vi "property_contour_interval_read.vi"(4 "error in (no error)":errorcluster, 6 "Container State":T29, 7 "Display State In":T1={"Graph Properties"={"Projection Mode"=enum."Orthographic", "View Direction"=enum."Towards X-Y Plane", "Plot Area Color"=0, "Fast Draw"=FALSE, "X-Y"=FALSE, "Y-Z"=FALSE, "X-Z"=FALSE, "Lighting"=FALSE, "Refnum Queue"=refnum}, "Plot/Axes/Cursor Properties"={"Plot Properties Array"=[{"Projection Properties"={"Draw XY"=FALSE, "Draw YZ"=FALSE, "Draw XZ"=FALSE}, "Surface Properties"={"Draw surface"=TRUE, "Opacity"=1.0, "Shading"=TRUE, "Specular"=100, "Color Map"=[], "Interpolate Color"=TRUE, "Absolute Colormap"=TRUE}, "Contour Properties"={"Contour color"=0, "Axis"=enum."X", "Draw contour"=FALSE, "Antialias"=FALSE, "Line Width"=1.0, "Contour Line Style"=enum."Solid", "Mode"=enum."Levels", "Levels"=5.0, "Intervals"=1.0, "Anchored At"=0.0, "Anchored"=FALSE, "Level List"=[]}, "Normal Properties"={"Normal color"=0, "Normal Length"=0.0, "Normal Width"=0.0, "Draw Normal"=FALSE, "Antialiasing"=FALSE}, "Points/Lines Properties"={"Color"=0, "Antialiasing"=FALSE, "Point Size"=0.0, "Points / Lines"=enum."None", "Point Style"=enum."Point", "Line Style"=enum."Solid", "Line Width"=0.0}, "Plot ID"=0, "Coordinate System"=enum."Cartesian"}], "Value Pair Properties"={"X Value Pairs"={"Data Array"=[], "Show ticks"=FALSE, "Show grid lines"=FALSE, "Labels"=enum."Value"}, "Y Value Pairs"={"Data Array"=[], "Show ticks"=FALSE, "Show grid lines"=FALSE, "Labels"=enum."Value"}, "Z Value Pairs"={"Data Array"=[], "Show ticks"=FALSE, "Show grid lines"=FALSE, "Labels"=enum."Value"}}, "Axes Properties"={"Grid  Properties"={"Grid Visible"={"Draw X-grid"=FALSE, "Draw Y-grid"=FALSE, "Draw Z-grid"=FALSE}, "Grid Color"={"Color X"=0, "Color Y"=0, "Color Z"=0}}, "Ticks Properties"={"Minor Count"={"X"=0, "Y"=0, "Z"=0}, "Major Count"={"X"=0, "Y"=0, "Z"=0}, "Major Ticks Visible"={"X"=FALSE, "Y"=FALSE, "Z"=FALSE}, "Minor Ticks Visible"={"X"=FALSE, "Y"=FALSE, "Z"=FALSE}, "Tick Color"={"Color X"=0, "Color Y"=0, "Color Z"=0}}, "from/to cluster"={"X"={"Min"=0.0, "Max"=0.0}, "Y"={"Min"=0.0, "Max"=0.0}, "Z"={"Min"=0.0, "Max"=0.0}, "Amplitude"={"Min"=0.0, "Max"=0.0}}, "Caption Properties"={"Show Captions"={"Show X Caption"=FALSE, "Show Z Caption"=FALSE, "Show Y Caption"=FALSE, "Show Opposite X Caption"=FALSE, "Show Opposite Y Caption"=FALSE, "Show Opposite Z Caption"=FALSE}, "Captions"={"Caption X"="", "Caption Y"="", "Caption Z"=""}, "Caption Color"={"Color X"=0, "Color Y"=0, "Color Z"=0}, "Caption Font Size"={"Font Size X"=0, "Font Size Y"=0, "Font Size Z"=0}}, "Labels Properties"={"Label Visible"={"Show X Labels"=FALSE, "Show Y Labels"=FALSE, "Show Z Labels"=FALSE, "Show Opposite X Labels"=FALSE, "Show Opposite Y Labels"=FALSE, "Show Opposite Z Labels"=FALSE}, "Label Color"={"Color X"=0, "Color Y"=0, "Color Z"=0}, "Label Font Size"={"Font Size X"=0, "Font Size Y"=0, "Font Size Z"=0}}, "Auto Range On"={"X"=FALSE, "Y"=FALSE, "Z"=FALSE}}, "Cursor Properties Array"=[], "Format strings"={"XAxis"="", "YAxis"="", "ZAxis"=""}, "Lighting Properties"={"Brightness"=0, "Focus"=0.0, "Linear Attenuation"=0.0, "Quadratic Attenuation"=0.0}, "Lights"=[]}, "Active Plot"=0, "Active Axis"=0, "Active Cursor"=0, "Disable Updates"=FALSE}) -> (0 "error out":errorcluster, 2 "Value":sgl, 3 "Display State Out":T1={"Graph Properties"={"Projection Mode"=enum."Orthographic", "View Direction"=enum."Towards X-Y Plane", "Plot Area Color"=0, "Fast Draw"=FALSE, "X-Y"=FALSE, "Y-Z"=FALSE, "X-Z"=FALSE, "Lighting"=FALSE, "Refnum Queue"=refnum}, "Plot/Axes/Cursor Properties"={"Plot Properties Array"=[{"Projection Properties"={"Draw XY"=FALSE, "Draw YZ"=FALSE, "Draw XZ"=FALSE}, "Surface Properties"={"Draw surface"=TRUE, "Opacity"=1.0, "Shading"=TRUE, "Specular"=100, "Color Map"=[], "Interpolate Color"=TRUE, "Absolute Colormap"=TRUE}, "Contour Properties"={"Contour color"=0, "Axis"=enum."X", "Draw contour"=FALSE, "Antialias"=FALSE, "Line Width"=1.0, "Contour Line Style"=enum."Solid", "Mode"=enum."Levels", "Levels"=5.0, "Intervals"=1.0, "Anchored At"=0.0, "Anchored"=FALSE, "Level List"=[]}, "Normal Properties"={"Normal color"=0, "Normal Length"=0.0, "Normal Width"=0.0, "Draw Normal"=FALSE, "Antialiasing"=FALSE}, "Points/Lines Properties"={"Color"=0, "Antialiasing"=FALSE, "Point Size"=0.0, "Points / Lines"=enum."None", "Point Style"=enum."Point", "Line Style"=enum."Solid", "Line Width"=0.0}, "Plot ID"=0, "Coordinate System"=enum."Cartesian"}], "Value Pair Properties"={"X Value Pairs"={"Data Array"=[], "Show ticks"=FALSE, "Show grid lines"=FALSE, "Labels"=enum."Value"}, "Y Value Pairs"={"Data Array"=[], "Show ticks"=FALSE, "Show grid lines"=FALSE, "Labels"=enum."Value"}, "Z Value Pairs"={"Data Array"=[], "Show ticks"=FALSE, "Show grid lines"=FALSE, "Labels"=enum."Value"}}, "Axes Properties"={"Grid  Properties"={"Grid Visible"={"Draw X-grid"=FALSE, "Draw Y-grid"=FALSE, "Draw Z-grid"=FALSE}, "Grid Color"={"Color X"=0, "Color Y"=0, "Color Z"=0}}, "Ticks Properties"={"Minor Count"={"X"=0, "Y"=0, "Z"=0}, "Major Count"={"X"=0, "Y"=0, "Z"=0}, "Major Ticks Visible"={"X"=FALSE, "Y"=FALSE, "Z"=FALSE}, "Minor Ticks Visible"={"X"=FALSE, "Y"=FALSE, "Z"=FALSE}, "Tick Color"={"Color X"=0, "Color Y"=0, "Color Z"=0}}, "from/to cluster"={"X"={"Min"=0.0, "Max"=0.0}, "Y"={"Min"=0.0, "Max"=0.0}, "Z"={"Min"=0.0, "Max"=0.0}, "Amplitude"={"Min"=0.0, "Max"=0.0}}, "Caption Properties"={"Show Captions"={"Show X Caption"=FALSE, "Show Z Caption"=FALSE, "Show Y Caption"=FALSE, "Show Opposite X Caption"=FALSE, "Show Opposite Y Caption"=FALSE, "Show Opposite Z Caption"=FALSE}, "Captions"={"Caption X"="", "Caption Y"="", "Caption Z"=""}, "Caption Color"={"Color X"=0, "Color Y"=0, "Color Z"=0}, "Caption Font Size"={"Font Size X"=0, "Font Size Y"=0, "Font Size Z"=0}}, "Labels Properties"={"Label Visible"={"Show X Labels"=FALSE, "Show Y Labels"=FALSE, "Show Z Labels"=FALSE, "Show Opposite X Labels"=FALSE, "Show Opposite Y Labels"=FALSE, "Show Opposite Z Labels"=FALSE}, "Label Color"={"Color X"=0, "Color Y"=0, "Color Z"=0}, "Label Font Size"={"Font Size X"=0, "Font Size Y"=0, "Font Size Z"=0}}, "Auto Range On"={"X"=FALSE, "Y"=FALSE, "Z"=FALSE}}, "Cursor Properties Array"=[], "Format strings"={"XAxis"="", "YAxis"="", "ZAxis"=""}, "Lighting Properties"={"Brightness"=0, "Focus"=0.0, "Linear Attenuation"=0.0, "Quadratic Attenuation"=0.0}, "Lights"=[]}, "Active Plot"=0, "Active Axis"=0, "Active Cursor"=0, "Disable Updates"=FALSE})   [LabVIEW 2020, in "3DPC_SurfacePlot.xctl"]
uses:
  <vilib>/Native 3D Graph/xcontrol/3DPC_SurfacePlot.xctl
  <vilib>/_xctls/Container State.ctl
  <vilib>/Native 3D Graph/xcontrol/State.ctl
  <vilib>/Native 3D Graph/typedefs/prop_graph.ctl
  <vilib>/Native 3D Graph/typedefs/all_non_graph_prop.ctl
  <vilib>/Native 3D Graph/typedefs/prop_plot_all_array.ctl
  <vilib>/Native 3D Graph/typedefs/prop_plot_all.ctl
  <vilib>/Native 3D Graph/typedefs/prop_plot_projection.ctl
  <vilib>/Native 3D Graph/typedefs/prop_plot_surface.ctl
  <vilib>/Native 3D Graph/typedefs/prop_plot_contour.ctl
  <vilib>/Native 3D Graph/typedefs/prop_plot_normal.ctl
  <vilib>/Native 3D Graph/typedefs/prop_plot_point_line.ctl
  <vilib>/Native 3D Graph/typedefs/prop_value_pair_all.ctl
  <vilib>/Native 3D Graph/typedefs/prop_value_pair_1d.ctl
  <vilib>/Native 3D Graph/typedefs/prop_axes_all.ctl
  <vilib>/Native 3D Graph/typedefs/prop_axes_grid.ctl
  <vilib>/Native 3D Graph/typedefs/prop_axes_ticks.ctl
  <vilib>/Native 3D Graph/typedefs/range_cluster.ctl
  <vilib>/Native 3D Graph/typedefs/min_max.ctl
  <vilib>/Native 3D Graph/typedefs/prop_axes_captions.ctl
  <vilib>/Native 3D Graph/typedefs/prop_axes_labels.ctl
  <vilib>/Native 3D Graph/typedefs/prop_axes_autorange.ctl
  <vilib>/Native 3D Graph/typedefs/prop_cursor_all_array.ctl
  <vilib>/Native 3D Graph/typedefs/prop_cursor_point.ctl
  <vilib>/Native 3D Graph/typedefs/prop_cursor_position.ctl
  <vilib>/Native 3D Graph/typedefs/prop_cursor_line.ctl
  <vilib>/Native 3D Graph/typedefs/prop_cursor_plane.ctl
  <vilib>/Native 3D Graph/typedefs/prop_cursor_text.ctl
  <vilib>/Native 3D Graph/typedefs/prop_format.ctl
  <vilib>/Native 3D Graph/typedefs/prop_lighting.ctl
  <vilib>/_xctls/XControlSupport.lvlib
panel:
  # "Replace the Value Indicator below with an Indicator of desired type.\nDo not remove this Indicator or the others from the connector pane. \nDo not change the connector pane pattern.\nThe Value Indicator should always be the second terminal from top on the output side in the connector pane."
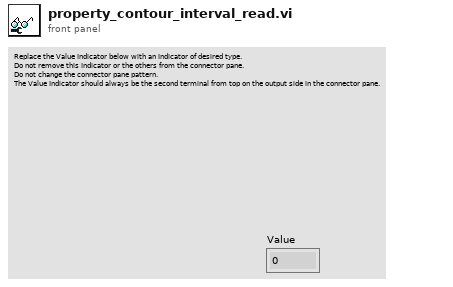
[diagram p1: front panel]
types:
  T1 = typedef "3DPC_SurfacePlot.xctl/State.ctl" = cluster{"Graph Properties":T2, "Plot/Axes/Cursor Properties":T3, "Active Plot":i32, "Active Axis":i32, "Active Cursor":i32, "Disable Updates":bool}
  T2 = typedef "3DPC_SurfacePlot.xctl/prop_graph.ctl" = cluster{"Projection Mode":enum16{"Orthographic", "Perspective"}, "View Direction":enum32{"Towards X-Y Plane", "Towards Y-Z Plane", "Towards X-Z Plane", "User Define"}, "Plot Area Color":u32, "Fast Draw":bool, "X-Y":bool, "Y-Z":bool, "X-Z":bool, "Lighting":bool, "Refnum Queue":refnum<queue>}
  T3 = typedef "3DPC_SurfacePlot.xctl/all_non_graph_prop.ctl" = cluster{"Plot Properties Array":T4, "Value Pair Properties":T11, "Axes Properties":T13, "Cursor Properties Array":T21, "Format strings":T27, "Lighting Properties":T28, "Lights":cluster{"Position":cluster{"X":sgl, "Y":sgl, "Z":sgl}, "Direction":cluster{"X":sgl, "Y":sgl, "Z":sgl}}[]}
  T4 = typedef "3DPC_SurfacePlot.xctl/prop_plot_all_array.ctl" = T5[]
  T5 = typedef "3DPC_SurfacePlot.xctl/prop_plot_all.ctl" = cluster{"Projection Properties":T6, "Surface Properties":T7, "Contour Properties":T8, "Normal Properties":T9, "Points/Lines Properties":T10, "Plot ID":i32, "Coordinate System":enum16{"Cartesian", "Cylindrical", "Spherical"}}
  T6 = typedef "3DPC_SurfacePlot.xctl/prop_plot_projection.ctl" = cluster{"Draw XY":bool, "Draw YZ":bool, "Draw XZ":bool}
  T7 = typedef "3DPC_SurfacePlot.xctl/prop_plot_surface.ctl" = cluster{"Draw surface":bool, "Opacity":dbl, "Shading":bool, "Specular":i32, "Color Map":cluster{dbl, u32}[], "Interpolate Color":bool, "Absolute Colormap":bool}
  T8 = typedef "3DPC_SurfacePlot.xctl/prop_plot_contour.ctl" = cluster{"Contour color":u32, "Axis":enum16{"X", "Y", "Z"}, "Draw contour":bool, "Antialias":bool, "Line Width":sgl, "Contour Line Style":enum16{"Solid", "Dash", "Dot", "Dash Dot"}, "Mode":enum16{"Levels", "Intervals", "Level List"}, "Levels":sgl, "Intervals":sgl, "Anchored At":sgl, "Anchored":bool, "Level List":dbl[]}
  T9 = typedef "3DPC_SurfacePlot.xctl/prop_plot_normal.ctl" = cluster{"Normal color":u32, "Normal Length":sgl, "Normal Width":sgl, "Draw Normal":bool, "Antialiasing":bool}
  T10 = typedef "3DPC_SurfacePlot.xctl/prop_plot_point_line.ctl" = cluster{"Color":u32, "Antialiasing":bool, "Point Size":sgl, "Points / Lines":enum16{"None", "Points", "Lines", "Both"}, "Point Style":enum16{"Point", "EmptySquare", "Asterisk", "Diamond", "EmptyCircle", "Circle", "X"}, "Line Style":enum16{"Solid", "Dash", "Dot", "Dash Dot"}, "Line Width":sgl}
  T11 = typedef "3DPC_SurfacePlot.xctl/prop_value_pair_all.ctl" = cluster{"X Value Pairs":cluster{"Data Array":cluster{"Value":sgl, "Index":i32, "Name":string}[], "Show ticks":bool, "Show grid lines":bool, "Labels":enum16{"Value", "None", "Name"}}, "Y Value Pairs":T12, "Z Value Pairs":T12}
  T12 = typedef "3DPC_SurfacePlot.xctl/prop_value_pair_1d.ctl" = cluster{"Data Array":cluster{"Value":sgl, "Index":i32, "Name":string}[], "Show ticks":bool, "Show grid lines":bool, "Labels":enum16{"Value", "None", "Name"}}
  T13 = typedef "3DPC_SurfacePlot.xctl/prop_axes_all.ctl" = cluster{"Grid  Properties":T14, "Ticks Properties":T15, "from/to cluster":T16, "Caption Properties":T18, "Labels Properties":T19, "Auto Range On":T20}
  T14 = typedef "3DPC_SurfacePlot.xctl/prop_axes_grid.ctl" = cluster{"Grid Visible":cluster{"Draw X-grid":bool, "Draw Y-grid":bool, "Draw Z-grid":bool}, "Grid Color":cluster{"Color X":u32, "Color Y":u32, "Color Z":u32}}
  T15 = typedef "3DPC_SurfacePlot.xctl/prop_axes_ticks.ctl" = cluster{"Minor Count":cluster{"X":i32, "Y":i32, "Z":i32}, "Major Count":cluster{"X":i32, "Y":i32, "Z":i32}, "Major Ticks Visible":cluster{"X":bool, "Y":bool, "Z":bool}, "Minor Ticks Visible":cluster{"X":bool, "Y":bool, "Z":bool}, "Tick Color":cluster{"Color X":u32, "Color Y":u32, "Color Z":u32}}
  T16 = typedef "3DPC_SurfacePlot.xctl/range_cluster.ctl" = cluster{"X":T17, "Y":T17, "Z":T17, "Amplitude":T17}
  T17 = typedef "3DPC_SurfacePlot.xctl/min_max.ctl" = cluster{"Min":sgl, "Max":sgl}
  T18 = typedef "3DPC_SurfacePlot.xctl/prop_axes_captions.ctl" = cluster{"Show Captions":cluster{"Show X Caption":bool, "Show Z Caption":bool, "Show Y Caption":bool, "Show Opposite X Caption":bool, "Show Opposite Y Caption":bool, "Show Opposite Z Caption":bool}, "Captions":cluster{"Caption X":string, "Caption Y":string, "Caption Z":string}, "Caption Color":cluster{"Color X":u32, "Color Y":u32, "Color Z":u32}, "Caption Font Size":cluster{"Font Size X":i16, "Font Size Y":i16, "Font Size Z":i16}}
  T19 = typedef "3DPC_SurfacePlot.xctl/prop_axes_labels.ctl" = cluster{"Label Visible":cluster{"Show X Labels":bool, "Show Y Labels":bool, "Show Z Labels":bool, "Show Opposite X Labels":bool, "Show Opposite Y Labels":bool, "Show Opposite Z Labels":bool}, "Label Color":cluster{"Color X":u32, "Color Y":u32, "Color Z":u32}, "Label Font Size":cluster{"Font Size X":i16, "Font Size Y":i16, "Font Size Z":i16}}
  T20 = typedef "3DPC_SurfacePlot.xctl/prop_axes_autorange.ctl" = cluster{"X":bool, "Y":bool, "Z":bool}
  T21 = typedef "3DPC_SurfacePlot.xctl/prop_cursor_all_array.ctl" = cluster{"Cursor Visible":bool, "Cursor Enable":bool, "Cursor Point":T22, "Cursor Position":T23, "Cursor Line":T24, "Cursor Plane":T25, "Cursor Name":string, "Cursor Text":T26}[]
  T22 = typedef "3DPC_SurfacePlot.xctl/prop_cursor_point.ctl" = cluster{"Point Color":u32, "Point Size":dbl, "Point Visible":bool}
  T23 = typedef "3DPC_SurfacePlot.xctl/prop_cursor_position.ctl" = cluster{"Position X":dbl, "Position Y":dbl, "Position Z":dbl, "Position Snap To":enum16{"Fixed", "Nearest Plot", "Snap to Plot"}, "Polsition Pick Plot":u16, "Position Column":i32, "Position Row":i32}
  T24 = typedef "3DPC_SurfacePlot.xctl/prop_cursor_line.ctl" = cluster{"Line Color":u32, "Line Width":dbl, "Line Visible":bool}
  T25 = typedef "3DPC_SurfacePlot.xctl/prop_cursor_plane.ctl" = cluster{"Plane Opacity":dbl, "Plane Color":u32, "Plane YZ":bool, "Plane XZ":bool, "Plane XY":bool}
  T26 = typedef "3DPC_SurfacePlot.xctl/prop_cursor_text.ctl" = cluster{"Cursor Name":string, "Font Size":i32, "Show Position":bool, "Show Name":bool, "Text Color":u32, "Back Color":u32, "Opacity":dbl}
  T27 = typedef "3DPC_SurfacePlot.xctl/prop_format.ctl" = cluster{"XAxis":string, "YAxis":string, "ZAxis":string}
  T28 = typedef "3DPC_SurfacePlot.xctl/prop_lighting.ctl" = cluster{"Brightness":i32, "Focus":dbl, "Linear Attenuation":dbl, "Quadratic Attenuation":dbl}
  T29 = typedef "XControlSupport.lvlib/Container State.ctl" = cluster{"Indicator?":bool, "Run Mode?":bool, " Refnum":refnum<vi>}
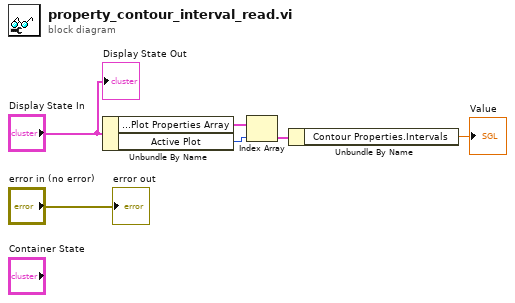
[diagram p0: block diagram]
diagram:
  n1 = Unbundle By Name("Display State In") -> ("Plot/Axes/Cursor Properties.Plot Properties Array"=w3:T4, "Active Plot"=w2:i32)
  n2 = Index Array(array=w3, index=w2) -> (element=w4:T5)
  n3 = Unbundle By Name(w4) -> ("Contour Properties.Intervals"=→"Value":sgl)
  "error out" <- "error in (no error)"
  "Display State Out" <- "Display State In"
